vi "SearchNode.vi"(8 "error in (no error)":errorcluster, 10 "LLNode in":refnum<data-value>, 11 "LLSearch in":refnum<class "LLSearch.lvclass">) -> (0 "error out":errorcluster, 1 "found":bool, 2 "LLNode out":refnum<data-value>, 3 "LLSearch out":refnum<class "LLSearch.lvclass">)   [LabVIEW 2009, in "LLSearch.lvclass"]
uses:
  LLSearch.lvclass
  LLNode/LLNode.lvclass
  Node/Node.lvclass
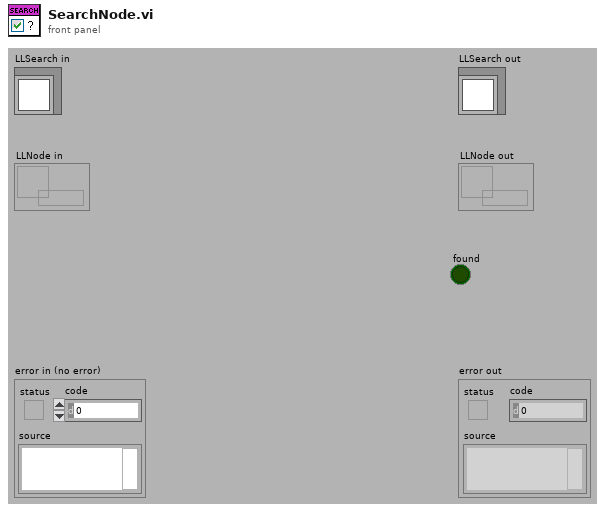
[diagram p1: front panel]
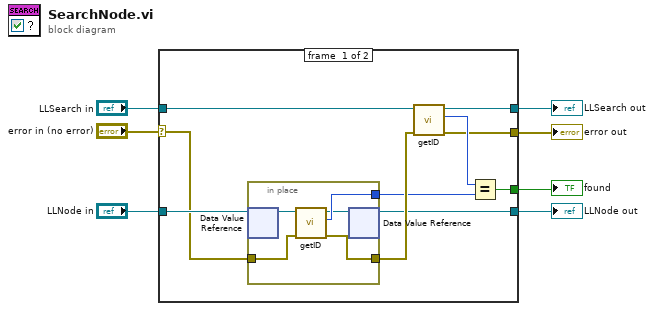
[diagram p0: block diagram]
diagram:
  n1 = case shown="No Error" "error in (no error)" {
    selector: "error in (no error)" -> [w11 w25]
    tunnel: [w9 w25] -> w6
    tunnel: [w14 w24] -> w4
    tunnel: "LLSearch in" -> [w15 w24]
    tunnel: "LLNode in" -> [w16 w23]
    tunnel: [w10 w23] -> w2
    tunnel: [w8 _] -> w1
    frame #0 {
      n2 = in-place {
        in-place-border: w11 -> [w21]
        in-place-border: [w18] -> w17
        in-place-border: [w20] -> w13
        n3 = in-place-dvr #1(w16) -> (w22:refnum<class "LLNode.lvclass">)  [unwired: 1 out]
        n4 = call "getID.vi"("error in (no error)"=w21, "Node in"=w22) -> ("error out"=w18:errorcluster, "ID"=w20:u32, "Node out"=w19:refnum<class "LLNode.lvclass">)  [unwired: 7 in]
        n5 = in-place-dvr #1(w19) -> (w10:refnum<data-value>)  [unwired: 1 out]
      }
      n6 = call "getID.vi"("error in (no error)"=w17, "LLSearch in"=w15) -> ("error out"=w9:errorcluster, "ID"=w12:u32, "LLSearch out"=w14:refnum<class "LLSearch.lvclass">)  [unwired: 7 in]
      n7 = Equal?(x=w12, y=w13) -> (x = y?=w8:bool)
    }
    frame #1 {
    }
  }
  "error out" <- w6
  "LLSearch out" <- w4
  "LLNode out" <- w2
  "found" <- w1
